vi "Write Session.TCPIP.MDNSBrowseTimeout.vi"(8 "error in (no error)":errorcluster, 10 "Session.TCPIP.MDNSBrowseTimeout":dbl, 11 "SLSC Remote in":refnum<class "SLSC Remote.lvclass">) -> (0 "error out":errorcluster, 3 "SLSC Remote out":refnum<class "SLSC Remote.lvclass">)   [LabVIEW 2015, in "SLSC Remote.lvclass"]
uses:
  SLSC Remote.lvclass
  <vilib>/rajsite/i3-json/JSON Generation/Create Value Files/Create Value - Numeric.vi
  <vilib>/rajsite/i3-json/i3-json.lvlib
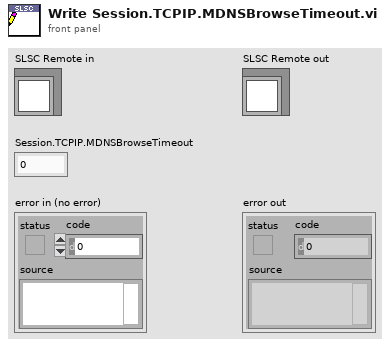
[diagram p1: front panel]
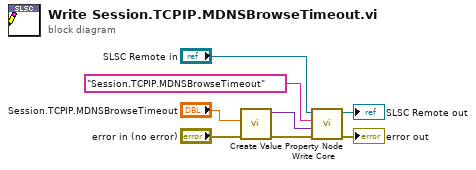
[diagram p0: block diagram]
diagram:
  n1 = call-poly <vilib>:"Create Value.vi"("error in (no error)"="error in (no error)", "Numeric"="Session.TCPIP.MDNSBrowseTimeout") -> ("error out"=w1:errorcluster, "JSON Tree"=w3:variant)  [unwired: 8 in]
  n2 = call "Property Node Write Core.vi"("error in (no error)"=w1, "value"=w3, "property"="Session.TCPIP.MDNSBrowseTimeout", "SLSC Remote in"="SLSC Remote in") -> ("error out"=→"error out":errorcluster, "SLSC Remote out"=→"SLSC Remote out":refnum<class "SLSC Remote.lvclass">)  [unwired: 6 in]
